vi "Read Pressure.vi"(8 "error in (no error)":errorcluster, 11 "Open Path Data in":refnum<class "Open Path Data.lvclass">) -> (0 "error out":errorcluster, 2 "Pressure":dbl, 3 "Open Path Data out":refnum<class "Open Path Data.lvclass">)   [LabVIEW 2019, in "Open Path Data.lvclass"]
uses:
  Open Path Data.lvclass
  Open Path Data.lvclass/Open Path Data.ctl
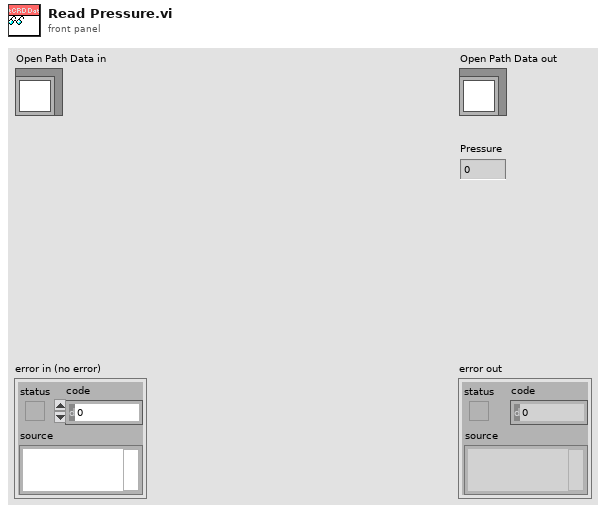
[diagram p1: front panel]
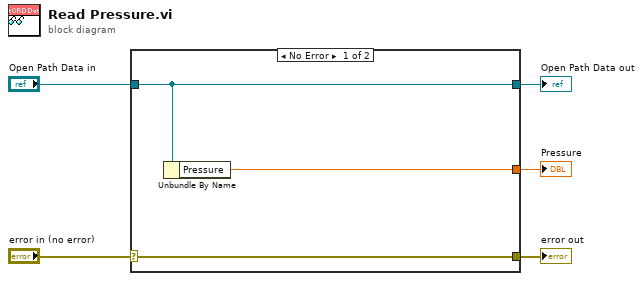
[diagram p0: block diagram]
diagram:
  n1 = case shown="No Error" "error in (no error)" {
    selector: "error in (no error)" -> [w8 w9]
    tunnel: [w8 w9] -> w4
    tunnel: [w7 w10] -> w2
    tunnel: "Open Path Data in" -> [w7 w10]
    tunnel: [w6 _] -> w1
    frame No Error {
      n2 = Unbundle By Name(w7) -> ("Pressure"=w6:dbl)
    }
    frame Error {
    }
  }
  "error out" <- w4
  "Open Path Data out" <- w2
  "Pressure" <- w1
